vi "string from the internet 1.vi"() -> ()   [LabVIEW 2010, in "Tank Robot.lvrbt"]
uses:
  Tank Robot.lvrbt
  <vilib>/NXT/NXT Controls/ConnectionType.ctl
  <vilib>/NXT/NXTIO Xnodes/AddressXNode/NXTIOAddress.xnode
  <vilib>/NXT/Subs/MotorXNode.DC Motor Type.ctl
  <vilib>/NXT/Subs/MotorXNode.2DCMotor.ctl
  <vilib>/NXT/NXTIO Xnodes/NXTIOXNode/NXTIO.xnode
  <vilib>/NXT/Subs/LVHSConnector.ctl
  <vilib>/NXT/NXTIO Xnodes/NXTIONodeSubVIs/TETRIX IO Move DC Motors.vi
panel:
  in  "Speed":dbl(slide) scale=0.0..100.0
  out "Drive Value":dbl
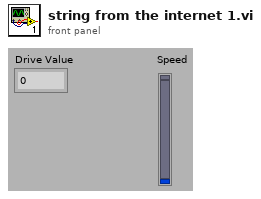
[diagram p1: front panel]
types:
  T1 = typedef "ConnectionType.ctl" = enum16{"Bluetooth", "USB", "WiFi"}
  T2 = typedef "LVHSConnector.ctl" = cluster{"Hardware":string, "Flattened String":string}
  T3 = typedef "MotorXNode.DC Motor Type.ctl" = enum16{"DC Motor"}
  T4 = cluster{"DC Motor":T3, "Address":i16, "Address":i16}
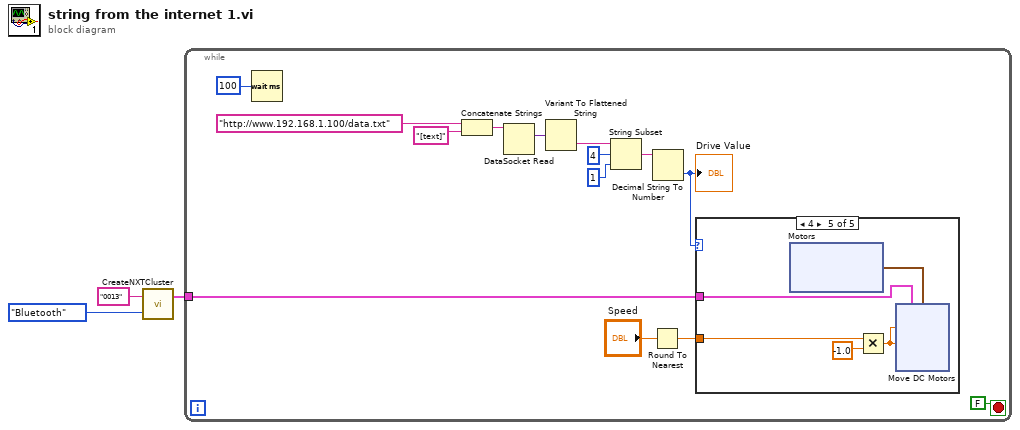
[diagram p0: block diagram]
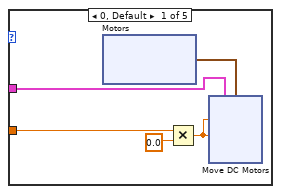
[diagram p2: hidden frame]
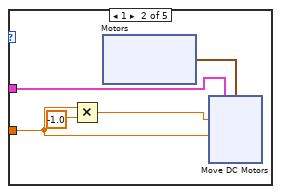
[diagram p3: hidden frame]
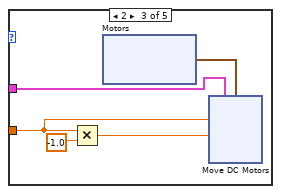
[diagram p4: hidden frame]
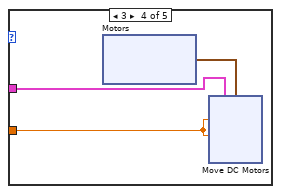
[diagram p5: hidden frame]
diagram:
  n1 = call <vilib>:"CreateNXTCluster.vi"("Connection Type"=ConnectionType."Bluetooth", "NXT name"="0013") -> ("NXT"=w3:T2)  [unwired: 2 in]
  n2 = while {
    tunnel: w3 -> [w4]
    stop <- FALSE stop-if-true
    n3 = Wait (ms)(milliseconds to wait=u32 100) -> ()  [unwired: 1 out]
    n4 = Concatenate Strings("http://www.192.168.1.100/data.txt" ("connection in"), "[text]" ("string")) -> (w15:string)
    n5 = DataSocket Read(11:w15) -> (2:w12:variant)  [unwired: 4 in, 6 out]
    n6 = Variant To Flattened String(Variant=w12) -> (data string=w8:string)  [unwired: 1 out]
    n7 = String Subset(string=w8, offset (0)=4, length (rest)=1 ("length (rest)")) -> (substring=w9:string)
    n8 = Round To Nearest(number="Speed") -> (nearest integer value=w5:dbl)
    n9 = Decimal String To Number(string=w9) -> (number=w7:i32)  [unwired: 2 in, 1 out]
    "Drive Value" <- w7
    n10 = case shown="4" w7 {
      tunnel: w5 -> [w21 w34 w50 w66 w82]
      tunnel: w4 -> [w18 w37 w52 w67 w83]
      frame 0, Default {
        n11 = xnode "Motors"() -> ("DC Motor"=w22:T4)
        n12 = Multiply(x=w21, y=0.0) -> (x*y=w19:dbl)
        n13 = xnode "Move DC Motors"("Power/Speed 2"=w19, "Power/Speed 1"=w19, "Motors"=w22, "NXT"=w18) -> ()  [unwired: 1 out]
      }
      frame 1 {
        n14 = Multiply(x=w34, y=-1.0) -> (x*y=w35:dbl)
        n15 = xnode "Motors"() -> ("DC Motor"=w38:T4)
        n16 = xnode "Move DC Motors"("Power/Speed 2"=w34, "Power/Speed 1"=w35, "Motors"=w38, "NXT"=w37) -> ()  [unwired: 1 out]
      }
      frame 2 {
        n17 = Multiply(x=w50, y=-1.0) -> (x*y=w51:dbl)
        n18 = xnode "Motors"() -> ("DC Motor"=w54:T4)
        n19 = xnode "Move DC Motors"("Power/Speed 2"=w51, "Power/Speed 1"=w50, "Motors"=w54, "NXT"=w52) -> ()  [unwired: 1 out]
      }
      frame 3 {
        n20 = xnode "Motors"() -> ("DC Motor"=w68:T4)
        n21 = xnode "Move DC Motors"("Power/Speed 2"=w66, "Power/Speed 1"=w66, "Motors"=w68, "NXT"=w67) -> ()  [unwired: 1 out]
      }
      frame 4 {
        n22 = xnode "Motors"() -> ("DC Motor"=w84:T4)
        n23 = Multiply(x=w82, y=-1.0) -> (x*y=w80:dbl)
        n24 = xnode "Move DC Motors"("Power/Speed 2"=w80, "Power/Speed 1"=w80, "Motors"=w84, "NXT"=w83) -> ()  [unwired: 1 out]
      }
    }
  }
